vi "CAN Frame to XNET Raw Frame.vi"(9 "timestamp":timestamp, 11 "CAN frame":T1 {"type" items=["CAN Data", "CAN Remote"]; "identifier" format="%.0x"}) -> (0 "error out":errorcluster, 2 "Raw Frame":u8[](array[numeric]))   [LabVIEW 2014]
uses:
  <vilib>/RioEmbeddedCAN/RioEmbeddedCAN.llb/CANFrameControl.ctl
  <vilib>/xnet/xnet.llb/XNET Frame CAN.ctl
  <vilib>/xnet/xnet.llb/XNET Frame Type CAN.ctl
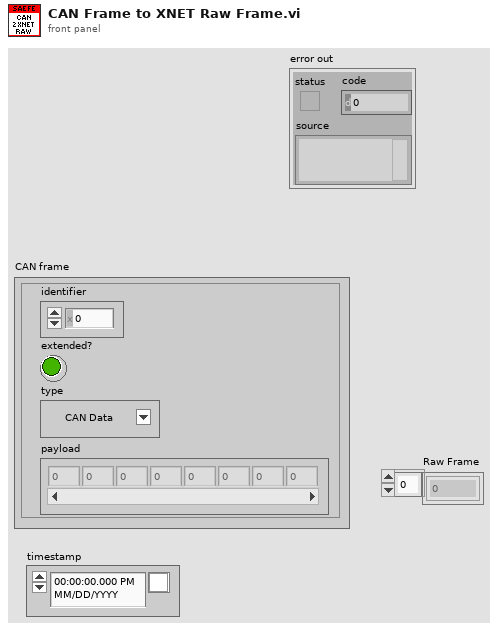
[diagram p1: front panel]
types:
  T1 = typedef "CANFrameControl.ctl" = cluster{"identifier":u32, "extended?":bool, "type":u8, "payload":u8[]}
  T2 = typedef "XNET Frame Type CAN.ctl" = u8
  T3 = typedef "XNET Frame CAN.ctl" = cluster{"timestamp":timestamp, "payload":u8[], "identifier":u32, "type":T2, "extended?":bool, "echo?":bool}
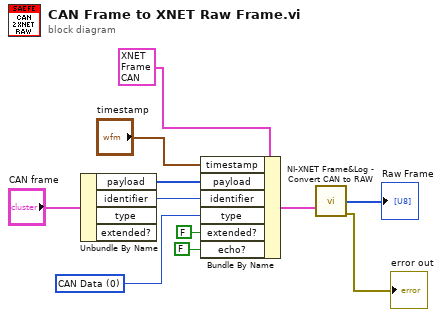
[diagram p0: block diagram]
diagram:
  w1 = T2 0 items=["CAN Data"=0, "CAN Remote"=1, "CAN Bus Error"=2, "Delay"=224, "Log Trigger"=225, "Start Trigger"=226] ("type")
  n1 = Unbundle By Name("CAN frame") -> ("payload"=w8:u8[], "identifier"=w7:u32)  [unwired: 2 out]
  n2 = Bundle By Name(cluster=T3 {"timestamp"=timestamp(0 s since 1904-01-01), "payload"=[], "identifier"=0, "type"=0, "extended?"=FALSE, "echo?"=FALSE} ("CAN frame"), "timestamp"="timestamp", "payload"=w8, "identifier"=w7, "type"=w1, "extended?"=FALSE, "echo?"=FALSE) -> (w5:T3)
  n3 = call "NI-XNET Frame&Log - Convert CAN to RAW.vi"("CAN frame"=w5) -> ("Raw Frame"=→"Raw Frame":u8[], "error out"=→"error out":errorcluster)  [unwired: 13 in]
